vi "DeleteData(SubVI).vi"(8 "Error In":errorcluster, 9 "String Array Out":string[](array[string]), 10 "CmbBox Refnum":refnum<vi>, 11 "Array in":refnum<vi>) -> (0 "Error Out":errorcluster)   [LabVIEW 2018]
uses:
  <vilib>/Utility/miscctls.llb/LVComboBoxStrsAndValuesArrayTypeDef.ctl
  CTL/Line.ctl
  Windows/Settings/View.ctl
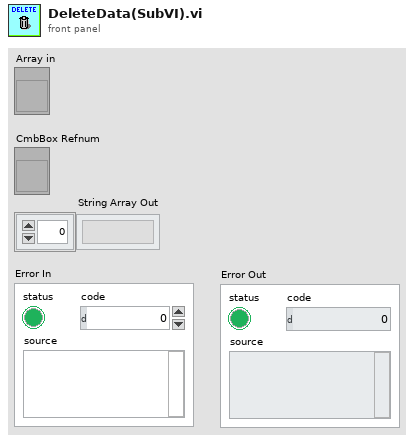
[diagram p1: front panel]
types:
  T1 = typedef "LVComboBoxStrsAndValuesArrayTypeDef.ctl" = cluster{"String":string, "Value":string}[]
  T2 = typedef "Line.ctl" = cluster{"Width":dbl, "Color":i64, "Array Oy":dbl[], "Array Ox":dbl[], "Name":string, "Plot Visible":T3}
  T3 = typedef "View.ctl" = bool
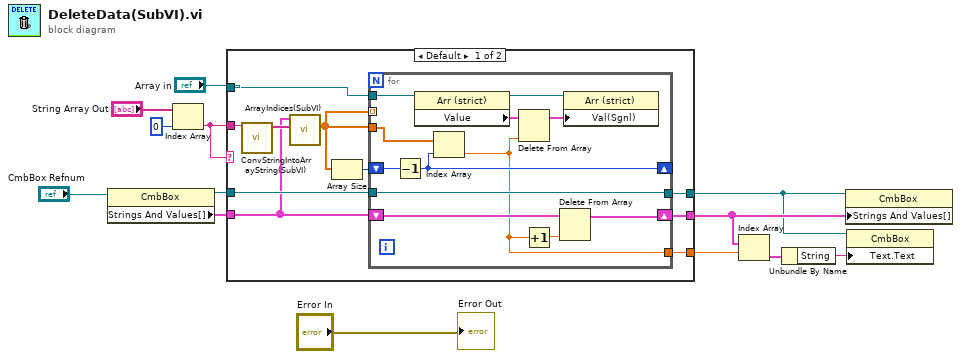
[diagram p0: block diagram]
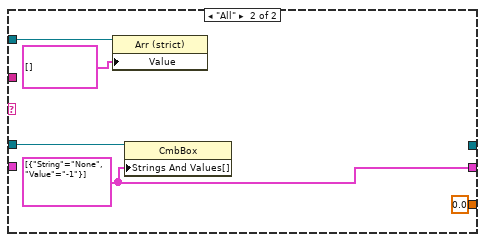
[diagram p2: hidden frame]
diagram:
  n1 = property on="Property Node" class="CmbBox"(reference="CmbBox Refnum") -> (reference out=w1:refnum<vi>, "Strings And Values[]"=w2:T1)  [unwired: 1 in, 1 out]
  n2 = Index Array(array="String Array Out", index=0) -> (element=w12:string)
  n3 = case shown="Default" w12 {
    tunnel: w12 -> [w20 _]
    tunnel: [w22 0.0 ("Index")] -> w10
    tunnel: "Array in" -> [w21 w39]
    tunnel: [w19 _] -> w3
    tunnel: [w18 w37] -> w4
    tunnel: w2 -> [w14 _]
    tunnel: w1 -> [w16 w36]
    frame Default {
      n4 = call "ConvStringIntoArrayString(SubVI).vi"("String In"=w20) -> ("Array String Out"=w17:string[])  [unwired: 9 in, 1 out]
      n5 = call "ArrayIndices(SubVI).vi"("Array In"=w17, "StringsAndValues[]"=w14) -> ("Array Out"=w15:dbl[])  [unwired: 8 in, 1 out]
      n6 = Array Size(array=w15) -> (size(s)=w23:i32)
      n7 = for {
        shift-right: [w33] -> _
        shift-left: w23 -> [w34]
        tunnel: w15 -> [w35]
        tunnel: [w24] -> w22
        tunnel: w21 -> [w29]
        shift-right: [w26] -> w18
        shift-left: w14 -> [w27]
        tunnel: [w25] -> w19
        tunnel: w16 -> [w25]
        tunnel: w15 -> [_] mode=indexing
        n8 = Decrement(x=w34) -> (x-1=w33:i32)
        n9 = property on="Property Node" class="Arr (strict)"(reference=w29) -> (reference out=w28:refnum<vi>, "Value"=w32:T2[])  [unwired: 1 in, 1 out]
        n10 = Index Array(array=w35, index=w33) -> (element=w24:dbl)
        n11 = Delete From Array(array=w32, index=w24) -> (array with subset deleted=w31:T2[])  [unwired: 1 in, 1 out]
        n12 = Increment(x=w24) -> (x+1=w30:dbl)
        n13 = Delete From Array(array=w27, index=w30) -> (array with subset deleted=w26:T1)  [unwired: 1 in, 1 out]
        n14 = property on="Property Node" class="Arr (strict)"(reference=w28, "Val(Sgnl)"=w31) -> ()  [unwired: 1 in, 2 out]
      }
    }
    frame "All" {
      w37 = T1 [{"String"="None", "Value"="-1"}] ("Strings And Values []")
      n15 = property on="Property Node" class="Arr (strict)"(reference=w39, "Value"=T2[] [] ("Value (Signaling)")) -> ()  [unwired: 1 in, 2 out]
      n16 = property on="Property Node" class="CmbBox"(reference=w36, "Strings And Values[]"=w37) -> ()  [unwired: 1 in, 2 out]
    }
  }
  n17 = Index Array(array=w4, index=w10) -> (element=w11:cluster{"String":string, "Value":string})
  n18 = Unbundle By Name(w11) -> ("String"=w13:string)
  n19 = property on="Property Node" class="CmbBox"(reference=w3, "Strings And Values[]"=w4) -> ()  [unwired: 1 in, 2 out]
  n20 = property on="Property Node" class="CmbBox"(reference=w3, "Text.Text"=w13) -> ()  [unwired: 1 in, 2 out]
  "Error Out" <- "Error In"
